vi "consecutive_true.vi"() -> ()   [LabVIEW 2018]
panel:
  out "s? t:f":u8
  in  "s":bool
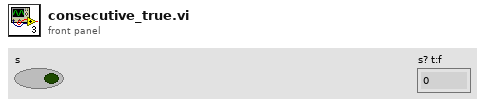
[diagram p1: front panel]
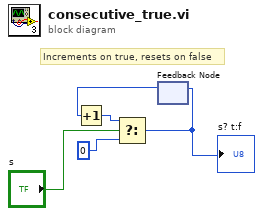
[diagram p0: block diagram]
diagram:
  # "Increments on true, resets on false"
  n1 = feedback #1() -> (w3:u8)  [unwired: 1 in]
  n2 = Increment(x=w3) -> (x+1=w2:u8)
  n3 = Select(t=w2, s="s", f=u8 0 ("t")) -> (s? t:f=w4:u8)
  "s? t:f" <- w4
  n4 = feedback-in #1(w4) -> ()
